vi "Read Info from File.vi"(8 "error in (no error)":errorcluster, 11 "VI File in":refnum<class "VI File.lvclass">) -> (0 "error out":errorcluster, 3 "VI File out":refnum<class "VI File.lvclass">)   [LabVIEW 2020, in "Save for Previous Version.lvlib" / "VI File.lvclass"]
uses:
  VI File.lvclass
  \\Mac\Home/JKI/GitHub/save-for-previous-labview-version/source/File/File.lvclass/File.lvclass
  \\Mac\Home/JKI/GitHub/save-for-previous-labview-version/source/LabVIEW File/LabVIEW File.lvclass
  File/File.lvclass/File.lvclass/File.ctl
  LabVIEW File/LabVIEW File.lvclass/LabVIEW File.ctl
  File/File.lvclass/Read Path.vi
  LabVIEW File/Write Version String.vi
  LabVIEW File/Write Version Number.vi
  LabVIEW File/LabVIEW File.lvclass
  VI File.lvclass/VI File.ctl
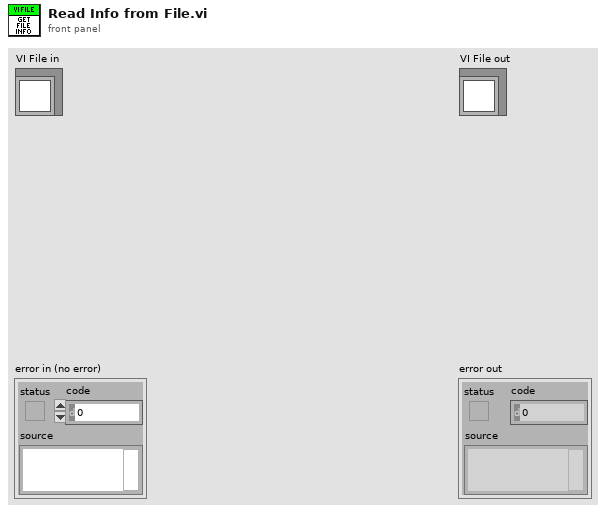
[diagram p1: front panel]
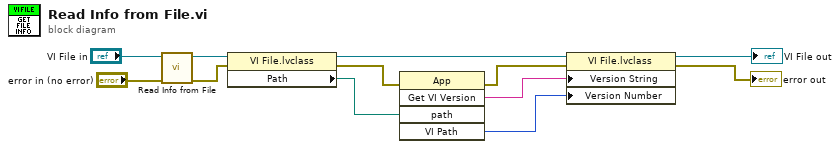
[diagram p0: block diagram]
diagram:
  n1 = call-parent "Read Info from File.vi"("error in (no error)"="error in (no error)", "LabVIEW File in"="VI File in") -> ("error out"=w4:errorcluster, "LabVIEW File out"=w6:refnum<class "VI File.lvclass">)  [unwired: 8 in]
  n2 = property class="VI File.lvclass"(reference=w6, error in=w4) -> (reference out=w5:refnum<class "VI File.lvclass">, error out=w2:errorcluster, "Path"=w3:path)
  n3 = invoke class="App" method="Get VI Version"(error in=w2, "path"=w3) -> (error out=w1:errorcluster, "GetVIVers"=w10:string, "VI Path"=w9:u32)  [unwired: 3 in, 2 out]
  n4 = property class="VI File.lvclass"(reference=w5, error in=w1, "Version String"=w10, "Version Number"=w9) -> (reference out=→"VI File out":refnum<class "VI File.lvclass">, error out=→"error out":errorcluster)
